vi "acc.vi"() -> ()   [LabVIEW 2019]
uses:
  <vilib>/Platform/TimedLoop/XDataNode/timing_clust.ctl
  <vilib>/Platform/TimedLoop/XDataNode/nitl_modes.ctl
  <vilib>/Platform/TimedLoop/XDataNode/wakeup.ctl
  <vilib>/myRIO/Instrument Drivers/Onboard IO/DIO/typedefs/DIO Reference.ctl
  <vilib>/myRIO/Common/Instrument Driver Framework/Utilities/typedefs/myRIO Generic Hardware Reference.ctl
  <vilib>/myRIO/Common/Instrument Driver Framework/Utilities/typedefs/Hardware Version Enum.ctl
  <vilib>/myRIO/Common/Instrument Driver Framework/Utilities/typedefs/myRIO v1.0 Reference.ctl
  <vilib>/myRIO/Common/Instrument Driver Framework/Utilities/typedefs/Generic FPGA Reference.ctl
  <vilib>/myRIO/Common/Instrument Driver Framework/myRIO v1.0/DIO/typedefs/DIO Channels List.ctl
  <vilib>/myRIO/Common/Instrument Driver Framework/myRIO v1.0/DIO/typedefs/DIO Channels Enum.ctl
  <vilib>/userDefined/High Color/nirio_resource_hc.ctl
  <vilib>/myRIO/Instrument Drivers/Onboard Devices/Accelerometer/typedefs/Accelerometer Reference.ctl
  <vilib>/myRIO/Common/Instrument Driver Framework/myRIO v1.0/Accelerometer/typedefs/Accelerometer Channels List.ctl
  <vilib>/myRIO/Common/Instrument Driver Framework/myRIO v1.0/Accelerometer/typedefs/Accelerometer Channels Enum.ctl
  <vilib>/myRIO/Common/Instrument Driver Framework/Utilities/vis/Is FPGA Ref Available.vi
  <vilib>/myRIO/Common/Instrument Driver Framework/myRIO v1.0/DIO/vis/myRIO v1.1 Open DIO.vi
  <vilib>/myRIO/Instrument Drivers/Onboard IO/DIO/vis/Read.vi
  <vilib>/myRIO/Common/Instrument Driver Framework/myRIO v1.0/Accelerometer/vis/myRIO v1.1 Open Accelerometer.vi
  <vilib>/myRIO/Instrument Drivers/Onboard Devices/Accelerometer/vis/Read.vi
  <vilib>/myRIO/Instrument Drivers/Onboard IO/DIO/vis/Write.vi
  <vilib>/myRIO/Common/Instrument Driver Framework/Utilities/vis/Validate Channels.vi
  <vilib>/myRIO/Common/Instrument Driver Framework/myRIO v1.0/DIO/vis/myRIO v1.0 Reserve DIO.vi
  <vilib>/myRIO/Common/Instrument Driver Framework/myRIO v1.0/Accelerometer/vis/myRIO v1.0 Reserve Accelerometer.vi
  <vilib>/myRIO/Common/Instrument Driver Framework/myRIO v1.0/Resource Manager/vis/myRIO v1.0 Reserve Channel List.vi
  <vilib>/myRIO/Common/Instrument Driver Framework/myRIO v1.0/DIO/vis/myRIO v1.0 Build MUX Configuration DIO.vi
  <vilib>/myRIO/Common/Instrument Driver Framework/myRIO v1.0/Accelerometer/vis/myRIO v1.0 Build MUX Configuration Accelerometer.vi
  <vilib>/myRIO/Common/Instrument Driver Framework/myRIO v1.0/Resource Manager/vis/myRIO v1.0 Reserve Channel.vi
  <vilib>/myRIO/Common/Instrument Driver Framework/myRIO v1.0/Resource Manager/vis/myRIO v1.0 Unreserve Channel.vi
  <vilib>/myRIO/Common/Instrument Driver Framework/myRIO v1.0/Resource Manager/vis/myRIO v1.0 Create Configuration List.vi
  <vilib>/myRIO/Common/Instrument Driver Framework/myRIO v1.0/Resource Manager/vis/myRIO v1.0 Build Mutex Name.vi
  <vilib>/Utility/VariantDataType/GetNumericInfo.vi
  <vilib>/Utility/error.llb/Error Cluster From Error Code.vi
  <vilib>/myRIO/Common/Instrument Driver Framework/myRIO v1.0/myRIO v1.1 Open.vi
  <vilib>/myRIO/Common/Instrument Driver Framework/Utilities/vis/IO Manager.vi
  <vilib>/myRIO/Common/Instrument Driver Framework/Utilities/vis/Configuration Manager.vi
  <vilib>/myRIO/Common/Instrument Driver Framework/myRIO v1.0/Resource Manager/vis/myRIO v1.0 Configure IO.vi
  <vilib>/myRIO/Common/Instrument Driver Framework/myRIO v1.0/myRIO v1.0 Close.vi
  <vilib>/myRIO/Common/Instrument Driver Framework/myRIO v1.0/DIO/vis/myRIO v1.0 Read DIO.vi
  <vilib>/myRIO/Common/Instrument Driver Framework/myRIO v1.0/Accelerometer/vis/myRIO v1.0 Get Scaling Constant Accelerometer.vi
  <vilib>/myRIO/Common/Instrument Driver Framework/myRIO v1.0/Accelerometer/vis/myRIO v1.0 Read Accelerometer.vi
  <vilib>/myRIO/Common/Instrument Driver Framework/myRIO v1.0/DIO/vis/myRIO v1.0 Write DIO.vi
  <vilib>/platform/TimedLoop/XDataNode/XDataNode.xnode
  <vilib>/myRIO/Express VI/Onboard Devices/Button/Button Express VI.xnode
  <vilib>/myRIO/Instrument Drivers/Onboard IO/DIO/vis/myRIO DIO Open.xnode
  <vilib>/myRIO/Express VI/Onboard Devices/Accelerometer/Accelerometer Express VI.xnode
  <vilib>/myRIO/Instrument Drivers/Onboard Devices/Accelerometer/vis/myRIO Accelerometer Open.xnode
  <vilib>/myRIO/Express VI/Onboard Devices/LED/LED Express VI.xnode
  <vilib>/Platform/TimedLoop/XDataNode/XDNodeRunTimeDep.lvlib
  <vilib>/myRIO/Instrument Drivers/Onboard IO/DIO/DIO.lvlib
  <vilib>/myRIO/Instrument Drivers/Onboard Devices/Accelerometer/Accelerometer.lvlib
panel:
  out "AngleTable":dbl[](array[numeric])
  in  "error in (no error)":errorcluster
  out "Axis":dbl[][](array[numeric])
  in  "stop 2":bool
  in  "stop":bool
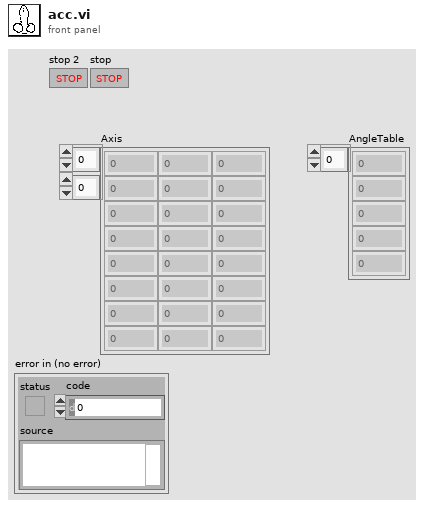
[diagram p1: front panel]
types:
  T1 = enum16{"open", "replace", "create", "open or create", "replace or create", "replace or create with confirmation"}
  T2 = typedef "DIO.lvlib/DIO Reference.ctl" = cluster{"myRIO Reference":T3, "DIO Channels List":T7}
  T3 = typedef "myRIO Generic Hardware Reference.ctl" = cluster{"myRIO Model":T4, "myRIO Hardware Reference":T5}
  T4 = typedef "Hardware Version Enum.ctl" = enum16{"Unknown", "myRIO-1900", "myRIO-1950", "roboRIO", "NI ELVIS RIO CM", "ELVIS III"}
  T5 = typedef "myRIO v1.0 Reference.ctl" = cluster{"Generic FPGA Reference":T6, "Allow multiple opens":bool}
  T6 = typedef "Generic FPGA Reference.ctl" = refnum<k20>
  T7 = typedef "DIO Channels List.ctl" = T8[]
  T8 = typedef "DIO Channels Enum.ctl" = enum16{"Not Connected", "C/DIO0", "C/DIO1", "C/DIO2", "C/DIO3", "C/DIO4", "C/DIO5", "C/DIO6", "C/DIO7", "A/DIO0", "A/DIO1", "A/DIO2", "A/DIO3", "A/DIO4", "A/DIO5", "A/DIO6", "A/DIO7", "A/DIO8", "A/DIO9", "A/DIO10", "A/DIO11", "A/DIO12", "A/DIO13", "A/DIO14", "A/DIO15", "A/DIO16", "A/DIO17", "A/DIO18", "A/DIO19", "B/DIO0", "B/DIO1", "B/DIO2", "B/DIO3", "B/DIO4", "B/DIO5", "B/DIO6", "B/DIO7", "B/DIO8", "B/DIO9", "B/DIO10", "B/DIO11", "B/DIO12", "B/DIO13", "B/DIO14", "B/DIO15", "B/DIO16", "B/DIO17", "B/DIO18", "B/DIO19", "LED0", "LED1", "LED2", "LED3", "Button0", "DIO/DIO0", "DIO/DIO1", "DIO/DIO2", "DIO/DIO3", "DIO/DIO4", "DIO/DIO5", "DIO/DIO6", "DIO/DIO7", "DIO/DIO8", "DIO/DIO9", "SPI/CS0", "SPI/CS1", "SPI/CS2", "SPI/CS3", "LED RADIO (Green)", "LED RADIO (Red)", "LED COMM (Green)", "LED COMM (Red)", "LED MODE (Green)", "LED MODE (Red)"}
  T9 = typedef "nirio_resource_hc.ctl" = tag
  T10 = typedef "Accelerometer.lvlib/Accelerometer Reference.ctl" = cluster{"myRIO Reference":T3, "Accelerometer Channels List":T11, "LSB Weight":dbl}
  T11 = typedef "Accelerometer Channels List.ctl" = T12[]
  T12 = typedef "Accelerometer Channels Enum.ctl" = enum16{"Not Connected", "X-Axis", "Y-Axis", "Z-Axis"}
  T13 = typedef "XDNodeRunTimeDep.lvlib/timing_clust.ctl" = cluster{"Expected End [f-1]":u64, "Actual End [f-1]":u64, "Finished Late? [f-1]":bool, "Expected End [i-1]":u64, "Actual End [i-1]":u64, "Finished Late? [i-1]":bool, "Expected Start [i]":u64, "Actual Start [i]":u64, "Expected Start [f]":u64, "Actual Start [f]":u64, "Source Name":string, "Structure Name":string, "Period":i64, "Deadline":i64, "Offset":i64, "Start":i64, "Priority":i32, "Timeout":i32, "Mode":T14, "Wakeup Reason":T15, "Error":errorcluster, "Source Type":string, "Secondary Source Type":string, "Global End Time":u64, "Global Start Time":u64, "Frame Duration":u64, "Iteration Duration":u64, "Assigned CPU":i32, "I/O Scan Engine Mode":u32}
  T14 = typedef "XDNodeRunTimeDep.lvlib/nitl_modes.ctl" = enum32{"No Change", "Process missed periods, maintain original phase", "Discard missed periods, maintain original phase", "Process missed periods, ignore original phase", "Discard missed periods, ignore original phase"}
  T15 = typedef "XDNodeRunTimeDep.lvlib/wakeup.ctl" = enum32{"Normal", "Aborted", "Asynchronous wakeup", "Timing source error", "Timed loop error", "Timeout"}
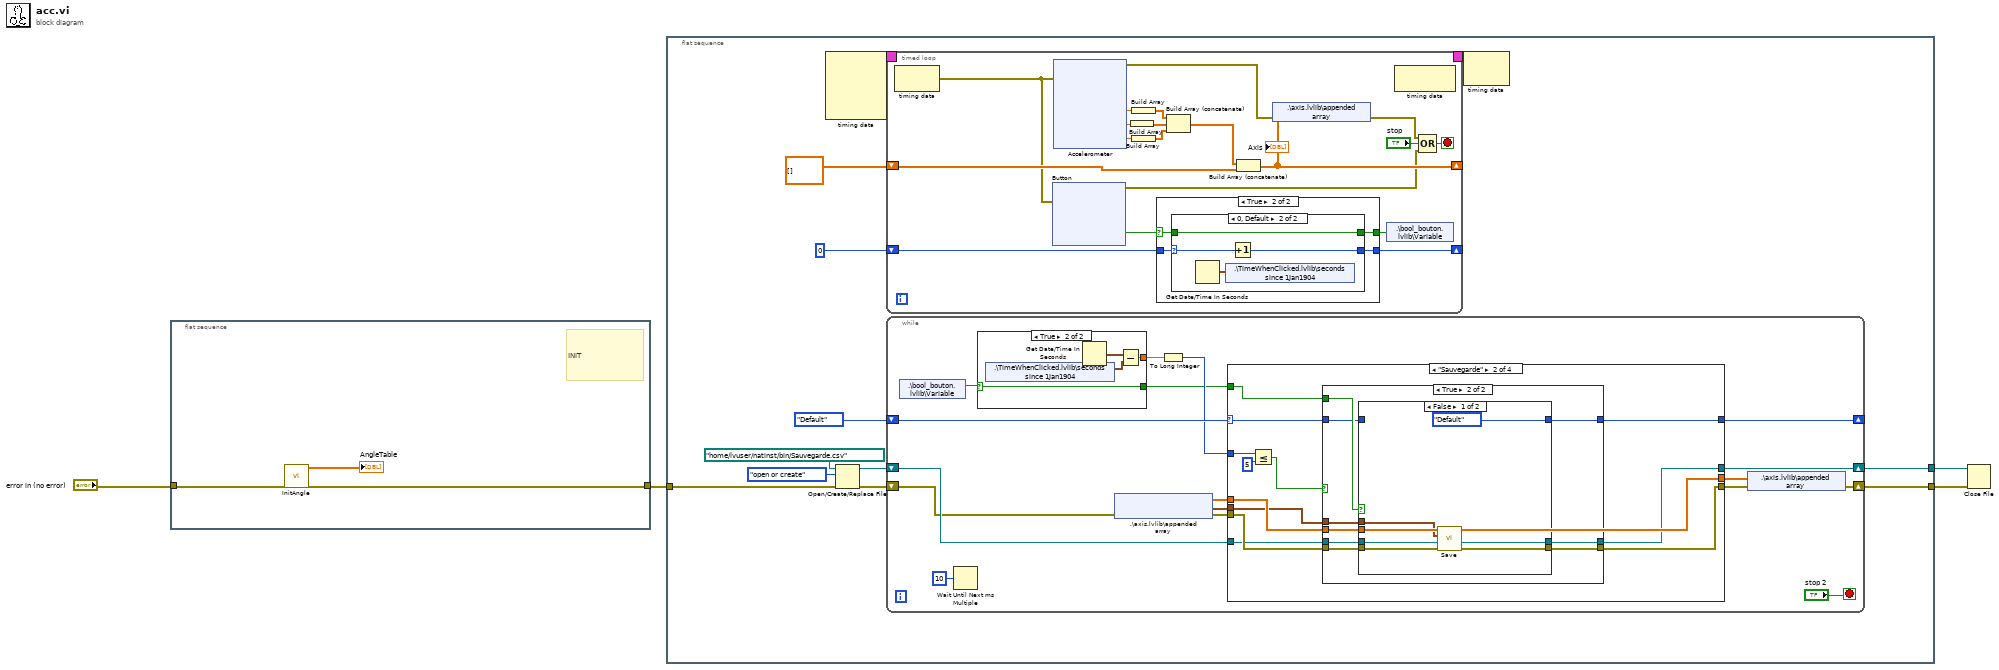
[diagram p0: block diagram]
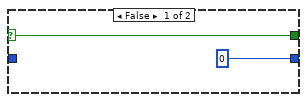
[diagram p2: hidden frame]
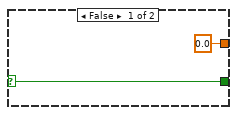
[diagram p4: hidden frame]
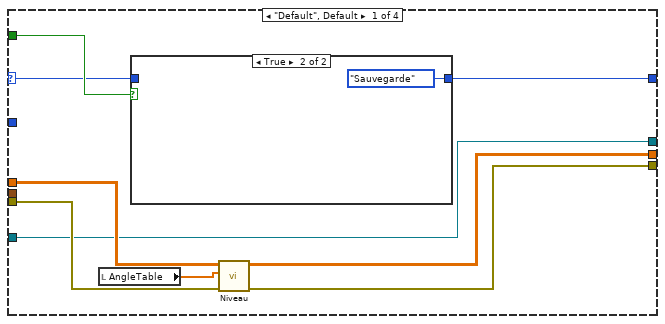
[diagram p5: hidden frame]
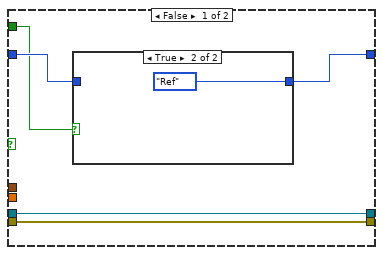
[diagram p7: hidden frame]
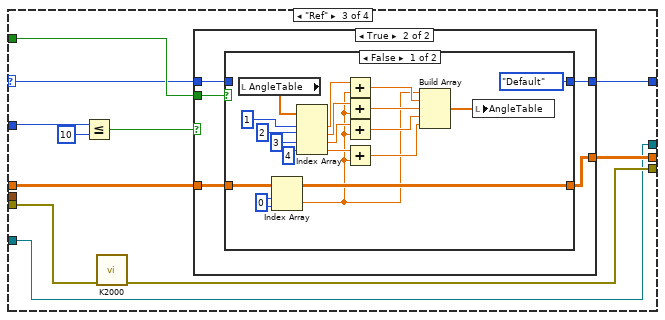
[diagram p10: hidden frame]
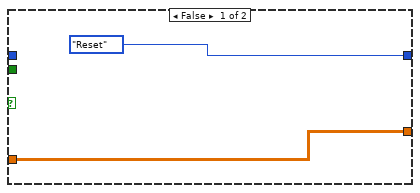
[diagram p11: hidden frame]
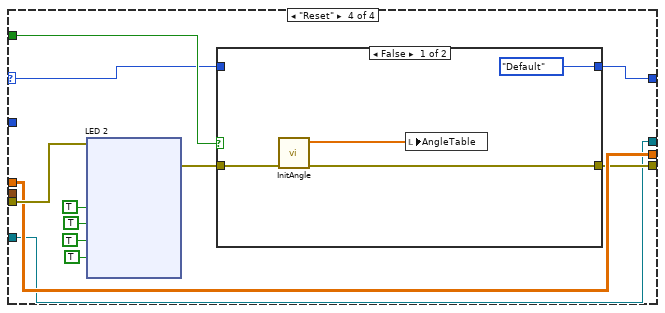
[diagram p13: hidden frame]
diagram:
  n1 = flat-sequence {
    tunnel: "error in (no error)" -> [w7]
    tunnel: [w6] -> w3
    frame #0 {
      # "INIT"
      n2 = call "InitAngle.vi"("error in (no error)"=w7) -> ("error out"=w6:errorcluster, "AngleTable"=→"AngleTable":dbl[])  [unwired: 9 in]
    }
  }
  n3 = flat-sequence {
    tunnel: w3 -> [w11]
    tunnel: [w10] -> w2
    tunnel: [w9] -> w1
    frame #0 {
      n4 = node-c288() -> (w19:T13)  [unwired: 4 in]
      n5 = Open/Create/Replace File(file path (use dialog)=path "/home/lvuser/natinst/bin/Sauvegarde.csv", error in=w11, operation (0:open)=T1."open or create") -> (refnum out=w8:refnum<file>, error out=w12:errorcluster)  [unwired: 3 in, 1 out]
      n6 = timed-loop {
        timing: w19 -> [_]
        timing-out: [_] -> w18
        shift-right: [w31] -> _
        shift-left: dbl[][] [] -> [w32]
        shift-right: [w27] -> _
        shift-left: 0 -> [w28]
        stop <- w22 stop-if-true
        n7 = node-c288() -> (w26:errorcluster)  [unwired: 1 in]
        n8 = xnode "Button"("error in (no error)"=w26) -> ("Value"=w29:bool, "error out"=w23:errorcluster)
        n9 = xnode "Accelerometer"("error in (no error)"=w26) -> ("Xaxis"=w20:dbl, "Yaxis"=w37:dbl, "Zaxis"=w38:dbl, "error out"=w30:errorcluster)
        n10 = Build Array(w37) -> (w35:dbl[])
        n11 = Build Array(w20) -> (w34:dbl[])
        n12 = Build Array(w38) -> (w36:dbl[])
        n13 = case shown="True" w29 {
          selector: w29 -> [w39 w42]
          tunnel: w28 -> [_ w44]
          tunnel: [0 w43] -> w27
          tunnel: [w39 w41] -> w21
          frame False {
          }
          frame True {
            n14 = case shown="0, Default" w44 {
              selector: w44 -> [w46 w50]
              tunnel: [w46 w49] -> w43
              tunnel: [w45 w48] -> w41
              tunnel: w42 -> [w45 w48]
              frame 1 {
              }
              frame 0, Default {
                n15 = Get Date/Time In Seconds() -> (seconds since 1Jan1904=w47:timestamp)
                n16 = shared-variable ".\\TimeWhenClicked.lvlib\\seconds since 1Jan1904"(w47) -> ()  [unwired: 1 in, 1 out]
                n17 = Increment(x=w50) -> (x+1=w49:i32)
              }
            }
          }
        }
        n18 = Build Array (concatenate)(w34, w35, w36) -> (w33:dbl[])
        n19 = Build Array (concatenate)(w33, w32) -> (w31:dbl[][])
        "Axis" <- w31
        n20 = shared-variable ".\\axis.lvlib\\appended array"(w31, error in=w30) -> (error out=w25:errorcluster)
        n21 = shared-variable ".\\bool_bouton.lvlib\\Variable"(w21) -> ()  [unwired: 1 in, 1 out]
        n22 = node-c288() -> ()  [unwired: 1 in, 1 out]
        n23 = Compound Arithmetic op=OR(w25, "stop", w23) -> (w22:bool)
      }
      n24 = while {
        shift-right: [w138] -> _
        shift-left: enum16{"Default", "Sauvegarde", "Ref", "Reset"}."Default" -> [w143]
        shift-right: [w144] -> w10
        shift-left: w12 -> [w131]
        shift-right: [w137] -> w9
        shift-left: w8 -> [w135]
        stop <- "stop 2" stop-if-true
        n25 = shared-variable ".\\bool_bouton.lvlib\\Variable"() -> (w130:bool)  [unwired: 1 in, 1 out]
        n26 = Wait Until Next ms Multiple(millisecond multiple=u32 10) -> ()  [unwired: 1 out]
        n27 = case shown="True" w130 {
          selector: w130 -> [w148 w152]
          tunnel: [w148 w152] -> w133
          tunnel: [0.0 w149] -> w132
          frame False {
          }
          frame True {
            n28 = shared-variable ".\\TimeWhenClicked.lvlib\\seconds since 1Jan1904"() -> (w150:timestamp)  [unwired: 1 in, 1 out]
            n29 = Get Date/Time In Seconds() -> (seconds since 1Jan1904=w151:timestamp)
            n30 = Subtract(x=w151, y=w150) -> (x-y=w149:dbl)
          }
        }
        n31 = shared-variable ".\\axis.lvlib\\appended array"(error in=w131) -> (w142:dbl[][], error out=w141:errorcluster, w136:timestamp)
        n32 = To Long Integer(number=w132) -> (32bit integer=w134:i32)
        n33 = case shown="\"Sauvegarde\"" w143 {
          selector: w143 -> [w155 w172 w207 w244]
          tunnel: w142 -> [w161 w169 w204 w243]
          tunnel: w141 -> [w160 w167 w205 w247]
          tunnel: [w159 w169 w203 w243] -> w140
          tunnel: [w158 w168 w206 w241] -> w139
          tunnel: w133 -> [w157 w170 w208 w246]
          tunnel: [w156 w173 w209 w245] -> w138
          tunnel: w134 -> [_ w175 w211 _]
          tunnel: [w153 w166 w202 w240] -> w137
          tunnel: w136 -> [_ w165 _ _]
          tunnel: w135 -> [w153 w164 w202 w240]
          frame "Default", Default {
            n34 = local read "AngleTable"() -> (w154:dbl[])
            n35 = case shown="True" w157 {
              tunnel: [w162 enum16{"Default", "Sauvegarde", "Ref", "Reset"}."Sauvegarde"] -> w156
              tunnel: w155 -> [w162 _]
              frame False {
              }
              frame True {
              }
            }
            n36 = call "Niveau.vi"("error in (no error)"=w160, "AngleTable"=w154, "Axis entrant"=w161) -> ("error out"=w158:errorcluster, "Axis sortant"=w159:dbl[][])  [unwired: 7 in]
          }
          frame "Sauvegarde" {
            n37 = Less Or Equal?(x=w175, y=5) -> (x <= y?=w171:bool)
            n38 = case shown="True" w171 {
              tunnel: [w180 w190] -> w173
              tunnel: w172 -> [w179 w189]
              tunnel: w170 -> [w178 w191]
              tunnel: w169 -> [_ w188]
              tunnel: w167 -> [w177 w187]
              tunnel: [w177 w186] -> w168
              tunnel: [w176 w185] -> w166
              tunnel: w165 -> [_ w184]
              tunnel: w164 -> [w176 w183]
              frame False {
                n39 = case shown="True" w178 {
                  tunnel: [w181 enum16{"Default", "Sauvegarde", "Ref", "Reset"}."Ref"] -> w180
                  tunnel: w179 -> [w181 _]
                  frame False {
                  }
                  frame True {
                  }
                }
              }
              frame True {
                n40 = case shown="False" w191 {
                  tunnel: [enum16{"Default", "Sauvegarde", "Ref", "Reset"}."Default" w201] -> w190
                  tunnel: w189 -> [_ w201]
                  tunnel: w188 -> [w197 _]
                  tunnel: w187 -> [w196 w200]
                  tunnel: [w195 w200] -> w186
                  tunnel: [w194 w199] -> w185
                  tunnel: w184 -> [w193 _]
                  tunnel: w183 -> [w192 w199]
                  frame False {
                    n41 = call "Save.vi"("error in (no error)"=w196, "refnum in"=w192, "time stamp"=w193, "array"=w197) -> ("error out"=w195:errorcluster, "refnum out"=w194:refnum<file>)  [unwired: 6 in]
                  }
                  frame True {
                  }
                }
              }
            }
          }
          frame "Ref" {
            n42 = Less Or Equal?(x=w211, y=10) -> (x <= y?=w210:bool)
            n43 = call "K2000.vi"("error constant"=w205) -> ("error constant 2"=w206:errorcluster)  [unwired: 10 in]
            n44 = case shown="True" w210 {
              tunnel: [enum16{"Default", "Sauvegarde", "Ref", "Reset"}."Reset" w218] -> w209
              tunnel: w208 -> [_ w219]
              tunnel: w207 -> [_ w217]
              tunnel: w204 -> [w213 w216]
              tunnel: [w213 w215] -> w203
              frame False {
              }
              frame True {
                n45 = case shown="False" w219 {
                  tunnel: [enum16{"Default", "Sauvegarde", "Ref", "Reset"}."Default" w239] -> w218
                  tunnel: w217 -> [_ w239]
                  tunnel: w216 -> [w235 w238]
                  tunnel: [w235 w238] -> w215
                  frame False {
                    w236 = 0 ("index (row)")
                    n46 = local read "AngleTable"() -> (w234:dbl[])
                    n47 = Index Array(array=w235, index (row)=w236, index (col)=w236) -> (element=w220:dbl)
                    n48 = Index Array(array=w234, index #1=1 ("index"), index #2=2 ("index"), index #3=3 ("index"), index #4=4 ("index")) -> (element #1=w229:dbl, element #2=w228:dbl, element #3=w227:dbl, element #4=w226:dbl)
                    n49 = Add(x=w229, y=w220) -> (x+y=w225:dbl)
                    n50 = Add(x=w228, y=w220) -> (x+y=w224:dbl)
                    n51 = Add(x=w227, y=w220) -> (x+y=w222:dbl)
                    n52 = Add(x=w226, y=w220) -> (x+y=w223:dbl)
                    n53 = Build Array(w220, w225, w224, w222, w223) -> (w221:dbl[])
                    n54 = local write "AngleTable"(w221) -> ()
                  }
                  frame True {
                  }
                }
              }
            }
          }
          frame "Reset" {
            n55 = xnode "LED 2"("L0"=TRUE, "L1"=TRUE ("L0"), "L2"=TRUE ("L0"), "L3"=TRUE ("L0"), "error in (no error)"=w247) -> ("error out"=w242:errorcluster)
            n56 = case shown="False" w246 {
              tunnel: [enum16{"Default", "Sauvegarde", "Ref", "Reset"}."Default" w257] -> w245
              tunnel: w244 -> [_ w257]
              tunnel: w242 -> [w254 w256]
              tunnel: [w253 w256] -> w241
              frame False {
                n57 = call "InitAngle.vi"("error in (no error)"=w254) -> ("error out"=w253:errorcluster, "AngleTable"=w252:dbl[])  [unwired: 9 in]
                n58 = local write "AngleTable"(w252) -> ()
              }
              frame True {
              }
            }
          }
        }
        n59 = shared-variable ".\\axis.lvlib\\appended array"(w140, error in=w139) -> (error out=w144:errorcluster)
      }
      n60 = node-c288(w18) -> ()  [unwired: 1 out]
    }
  }
  n61 = Close File(refnum=w1, error in=w2) -> ()  [unwired: 2 out]
